vi "AddTaskbarIcon.vi"(6 "hWnd (NULL)":T1, 7 "Callback Message\n(0 - NULL)":i32, 8 "error in (no error)":errorcluster, 9 "hIcon (NULL)":i32, 10 "uID (1)":i32=1, 11 "Tooltip Text (\"\")":string) -> (0 "error out":errorcluster)   [LabVIEW 2011]
uses:
  WinUSER/Windows/hWnd.ctl
  NOTIFYICON_OPERATIONS.ctl
  NOTIFYICONDATA.ctl
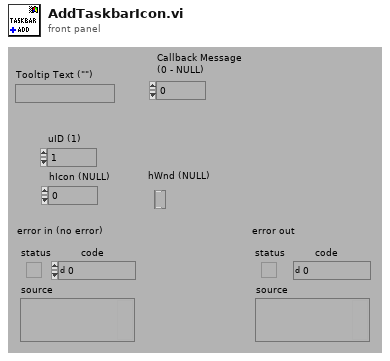
[diagram p1: front panel]
types:
  T1 = typedef "hWnd.ctl" = refnum<k1>
  T2 = typedef "NOTIFYICON_OPERATIONS.ctl" = enum16{"NIM_ADD", "NIM_MODIFY", "NIM_DELETE", "NIM_SETFOCUS", "NIM_SETVERSION"}
  T3 = typedef "NOTIFYICONDATA.ctl" = cluster{"cbSize":i32, "hWnd":i32, "uID":i32, "uFlags":i32, "uCallbackMessage":i32, "hIcon":i32, "szTip[64]":string}
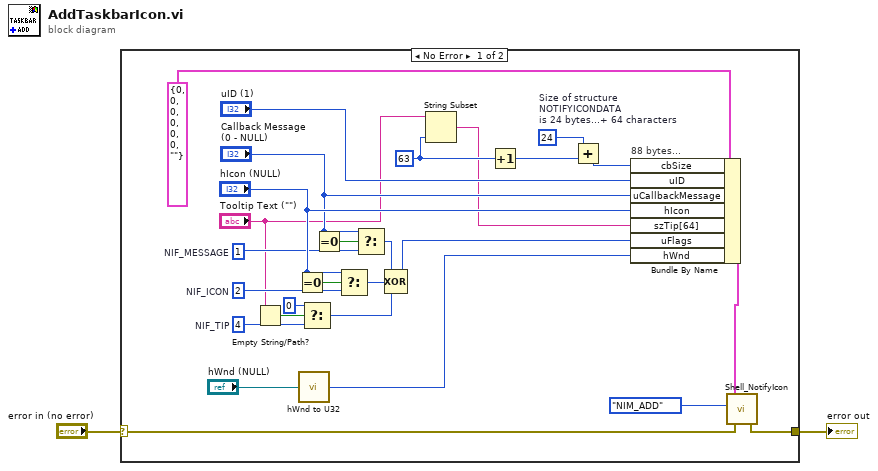
[diagram p0: block diagram]
diagram:
  n1 = case shown="No Error" "error in (no error)" {
    selector: "error in (no error)" -> [w5 w30]
    tunnel: [w15 w30] -> w1
    frame No Error {
      w8 = 63 ("length (rest)")
      w11 = 24  # Size of structure NOTIFYICONDATA is 24 bytes...+ 64 characters
      w17 = 1  # NIF_MESSAGE
      w21 = 2  # NIF_ICON
      w26 = 4  # NIF_TIP
      # "88 bytes..."
      n2 = Empty String/Path?(string/path="Tooltip Text (\"\")") -> (empty?=w28:bool)
      n3 = Equal To 0?(x="hIcon (NULL)") -> (x = 0?=w23:bool)
      n4 = call "hWnd to U32.vi"("hWnd"="hWnd (NULL)") -> ("hWnd"=w3:u32)  [unwired: 4 out]
      n5 = Select(t=0, s=w28, f=w26) -> (s? t:f=w25:i32)
      n6 = Equal To 0?(x="Callback Message\n(0 - NULL)") -> (x = 0?=w19:bool)
      n7 = Select(t="hIcon (NULL)", s=w23, f=w21) -> (s? t:f=w24:i32)
      n8 = Select(t="Callback Message\n(0 - NULL)", s=w19, f=w17) -> (s? t:f=w18:i32)
      n9 = Compound Arithmetic op=XOR(w18, w24, w25) -> (w16:i32)
      n10 = String Subset(string="Tooltip Text (\"\")", length (rest)=w8) -> (substring=w6:string)  [unwired: 1 out]
      n11 = Increment(x=w8) -> (x+1=w7:i32)
      n12 = Add(x=w11, y=w7) -> (x+y=w10:i32)
      n13 = Bundle By Name(cluster=T3 {"cbSize"=0, "hWnd"=0, "uID"=0, "uFlags"=0, "uCallbackMessage"=0, "hIcon"=0, "szTip[64]"=""} ("NOTIFYICONDATA"), "cbSize"=w10, "uID"="uID (1)", "uCallbackMessage"="Callback Message\n(0 - NULL)", "hIcon"="hIcon (NULL)", "szTip[64]"=w6, "uFlags"=w16, "hWnd"=w3) -> (w14:T3)
      n14 = call "Shell_NotifyIcon.vi"("error in (no error)"=w5, "Operation (NIF_ADD)"=NOTIFYICON_OPERATIONS."NIM_ADD", "NOTIFYICONDATA"=w14) -> ("error out"=w15:errorcluster)  [unwired: 4 out]
    }
    frame Error {
    }
  }
  "error out" <- w1
